vi "Error Query.vi"(7 "Add instrument error to error cluster (T)":bool=TRUE, 8 "error in (no error)":errorcluster, 11 "VISA resource name":refnum<visa-resource-name>) -> (0 "error out":errorcluster, 1 "Error Message(s)":string, 2 "Error":i32, 3 "VISA resource name out":refnum<visa-resource-name>)   [LabVIEW 2015, in "Rohde&Schwarz CMXP Base.lvlib"]
doc: "This VI reads <b>ALL</b> the errors from the instrument's error queue. It expects to read the errors in SCPI format (#,\"error message\").\nThese messages are <b>DELETED</b> from the error queue after reading.\n\nRemote-control command:\nSYSTem:ERRor?"
uses:
  <instrlib>/Rohde&Schwarz CMXP Base/Rohde&Schwarz CMXP Base.lvlib
  <instrlib>/Rohde&Schwarz CMXP Base/Private/rsidr_core.llb/rsidr_core.lvlib
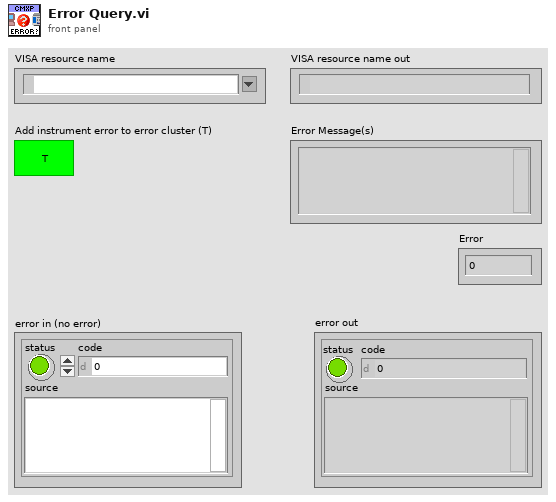
[diagram p1: front panel]
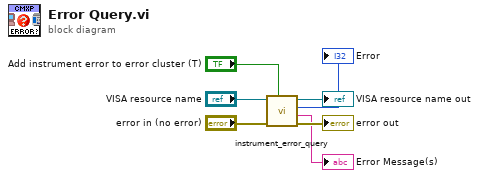
[diagram p0: block diagram]
diagram:
  n1 = call <instrlib>:"instrument_error_query.vi"("Add instrument error to error cluster (T)"="Add instrument error to error cluster (T)", "error in"="error in (no error)", "VISA resource name"="VISA resource name") -> ("error out"=→"error out":errorcluster, "Error Message(s) out"=→"Error Message(s)":string, "Error Code"=→"Error":i32, "VISA resource name out"=→"VISA resource name out":refnum<visa-resource-name>)  [unwired: 5 in]
